vi "Sort_Matrix_DBL.vi"(1 "Unsort array in":dbl[][](array[numeric])) -> (21 "Sorted array out":dbl[][](array[numeric]))   [LabVIEW 2025]
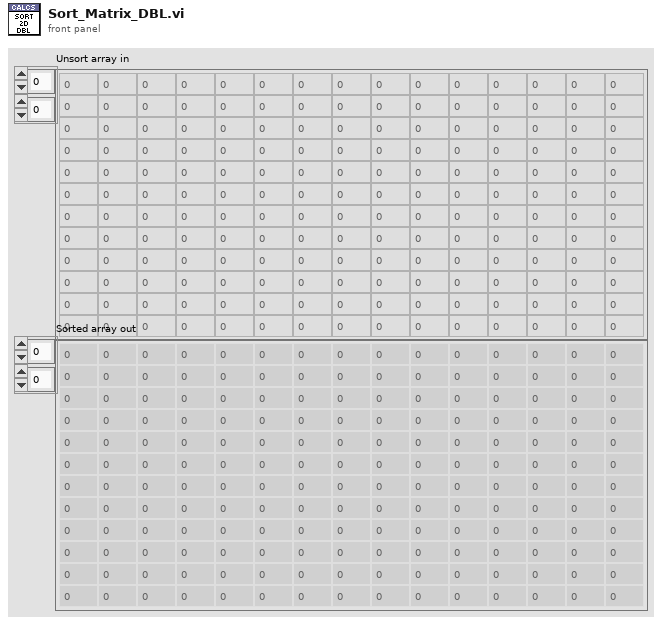
[diagram p1: front panel]
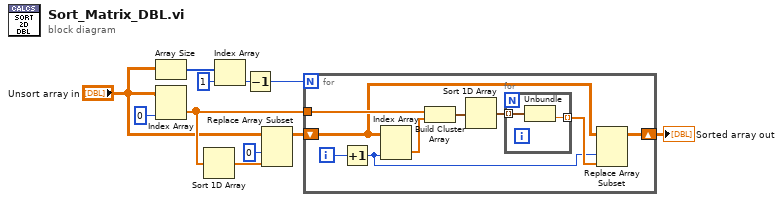
[diagram p0: block diagram]
diagram:
  n1 = Array Size(array="Unsort array in") -> (size(s)=w11:i32[])
  n2 = Index Array(array="Unsort array in", index (col)=0 ("index")) -> (element=w7:dbl[])  [unwired: 1 in]
  n3 = Sort 1D Array(array=w7) -> (sorted array=w5:dbl[])
  n4 = Index Array(array=w11, index=1) -> (element=w9:i32)
  n5 = Decrement(x=w9) -> (x-1=w8:i32)
  n6 = Replace Array Subset(array="Unsort array in", new element=w5, index (col)=0 ("index (row)")) -> (w4:dbl[][])  [unwired: 1 in]
  n7 = for {
    N: w8 -> [_]
    tunnel: w7 -> [w19]
    shift-right: [w13] -> w3
    shift-left: w4 -> [w15]
    i -> [w20]
    n8 = Increment(x=w20) -> (x+1=w12:i32)
    n9 = Index Array(array=w15, index (col)=w12) -> (element=w18:dbl[])  [unwired: 1 in]
    n10 = Build Cluster Array(w19, w18) -> (w17:cluster{"Numeric":dbl, "Numeric":dbl}[])
    n11 = Sort 1D Array(array=w17) -> (sorted array=w16:cluster{"Numeric":dbl, "Numeric":dbl}[])
    n12 = for {
      tunnel: w16 -> [w22] mode=indexing
      tunnel: [w21] -> w14 mode=indexing
      n13 = Unbundle(w22) -> ("Numeric"=w21:dbl)  [unwired: 1 out]
    }
    n14 = Replace Array Subset(array=w15, new element=w14, index (col)=w12) -> (w13:dbl[][])  [unwired: 1 in]
  }
  "Sorted array out" <- w3
